vi "Get PathName.vi"(8 "error in (no error)":errorcluster caption="错误输入（无错误）", 11 "Item输入":refnum<class "Item.lvclass">) -> (0 "error out":errorcluster caption="错误输出", 2 "PathName":string, 3 "Item输出":refnum<class "Item.lvclass">)   [LabVIEW 2013, in "Hierarchy Framework.lvlib" / "Item.lvclass"]
uses:
  Item.lvclass
  Item.lvclass/Item.ctl
  Generic/Generic.lvclass
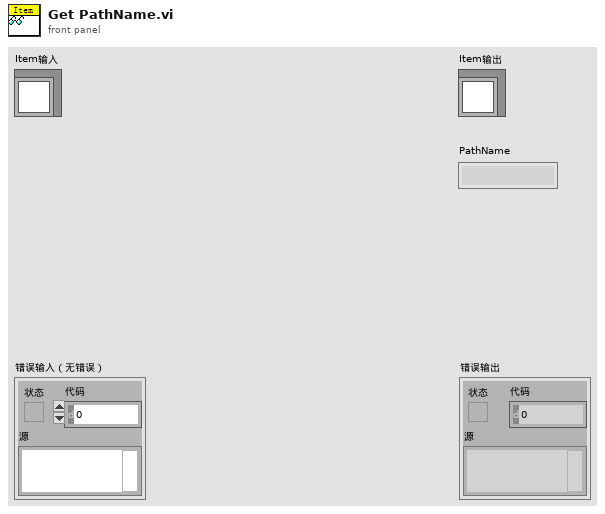
[diagram p1: front panel]
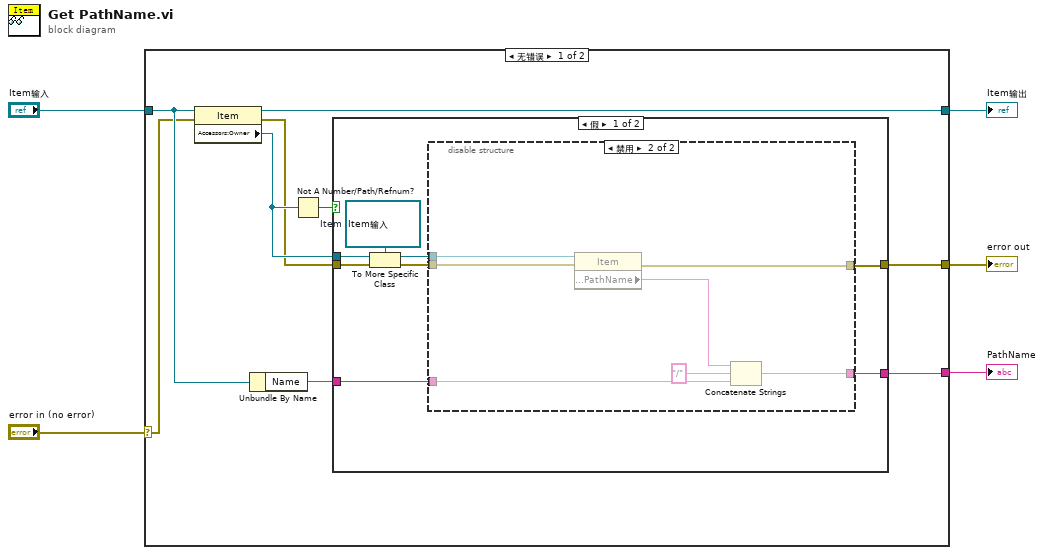
[diagram p0: block diagram]
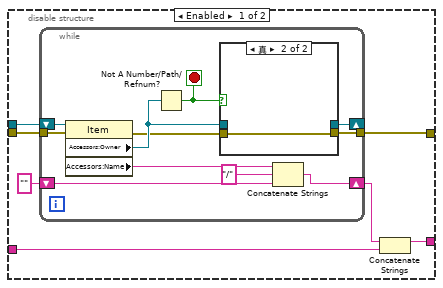
[diagram p2: hidden frame]
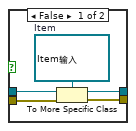
[diagram p3: hidden frame]
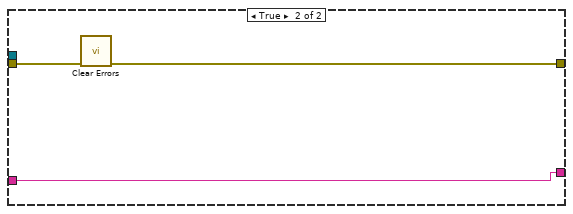
[diagram p4: hidden frame]
diagram:
  n1 = case shown="无错误" "error in (no error)" {
    selector: "error in (no error)" -> [w6 w57]
    tunnel: [w9 w57] -> w4
    tunnel: [w12 w58] -> w2
    tunnel: "Item输入" -> [w8 w58]
    tunnel: [w13 _] -> w1
    frame No Error {
      n2 = property class="Item"(reference=w8, error in=w6) -> (reference out=w12:refnum<class "Item.lvclass">, error out=w10:errorcluster, "Accessors:Owner"=w11:refnum<data-value>)
      n3 = Unbundle By Name(w8) -> ("Name"=w7:string)
      n4 = Not A Number/Path/Refnum?(number/path/refnum=w11) -> (NaN/Path/Refnum?=w14:bool)
      n5 = case shown="假" w14 {
        tunnel: w11 -> [w22 _]
        tunnel: [w15 w56] -> w13
        tunnel: w7 -> [w16 w56]
        tunnel: w10 -> [w20 w55]
        tunnel: [w17 w54] -> w9
        frame False {
          w21 = refnum<data-value> refnum  # Item
          n6 = To More Specific Class(target class=w21, reference=w22, error in=w20) -> (specific class reference=w19:refnum<data-value>, error out=w18:errorcluster)
          n7 = disable-structure shown="禁用" {
            disable-tunnel: w19 -> [w29 w53]
            disable-tunnel: w18 -> [w28 w52]
            disable-tunnel: [w26 w51] -> w17
            disable-tunnel: [w23 w47] -> w15
            disable-tunnel: w16 -> [w24 w49]
            frame Enabled {
              n8 = while {
                tunnel: w28 -> [w39]
                shift-right: [w37] -> _
                shift-left: w29 -> [w40]
                shift-right: [w35] -> w25
                shift-left: "" -> [w34]
                tunnel: [w32] -> w26
                stop <- w31 stop-if-true
                n9 = property class="Item"(reference=w40, error in=w39) -> (error out=w33:errorcluster, "Accessors:Owner"=w38:refnum<data-value>, "Accessors:Name"=w36:string)  [unwired: 1 out]
                n10 = Not A Number/Path/Refnum?(number/path/refnum=w38) -> (NaN/Path/Refnum?=w31:bool)
                n11 = case shown="真" w31 {
                  tunnel: w38 -> [w45 _]
                  tunnel: [w44 _] -> w37
                  tunnel: w33 -> [w43 w46]
                  tunnel: [w42 w46] -> w32
                  frame False {
                    w41 = refnum<data-value> refnum  # Item
                    n12 = To More Specific Class(target class=w41, reference=w45, error in=w43) -> (specific class reference=w44:refnum<data-value>, error out=w42:errorcluster)
                  }
                  frame True {
                  }
                }
                n13 = Concatenate Strings(w36, "/" ("字符串"), w34) -> (w35:string)
              }
              n14 = Concatenate Strings(w25, w24) -> (w23:string)
            }
            frame Disabled {
              n15 = property class="Item"(reference=w53, error in=w52) -> (error out=w51:errorcluster, "Accessors:PathName"=w50:string)  [unwired: 1 out]
              n16 = Concatenate Strings(w50, "/" ("字符串"), w49) -> (w47:string)
            }
          }
        }
        frame True {
          n17 = call <vilib>:"Clear Errors.vi"("error in (no error)"=w55) -> ("error out"=w54:errorcluster)  [unwired: 6 in]
        }
      }
    }
    frame Error {
    }
  }
  "error out" <- w4
  "Item输出" <- w2
  "PathName" <- w1
